vi "cost_complexity_pruning_path.vi"(8 "error in (no error)":errorcluster, 11 "Interface_cost_complexity_pruning_path in":refnum<class "Interface_cost_complexity_pruning_path.lvclass">) -> (0 "error out":errorcluster, 2 "out":cluster{"ccp_alphas":dbl[], "impurities":dbl[]}, 3 "Interface_cost_complexity_pruning_path out":refnum<class "Interface_cost_complexity_pruning_path.lvclass">)   [LabVIEW 2020, in "Interface_cost_complexity_pruning_path.lvclass"]
doc: "Compute the pruning path during Minimal Cost-Complexity Pruning."
uses:
  Interface_cost_complexity_pruning_path.lvclass
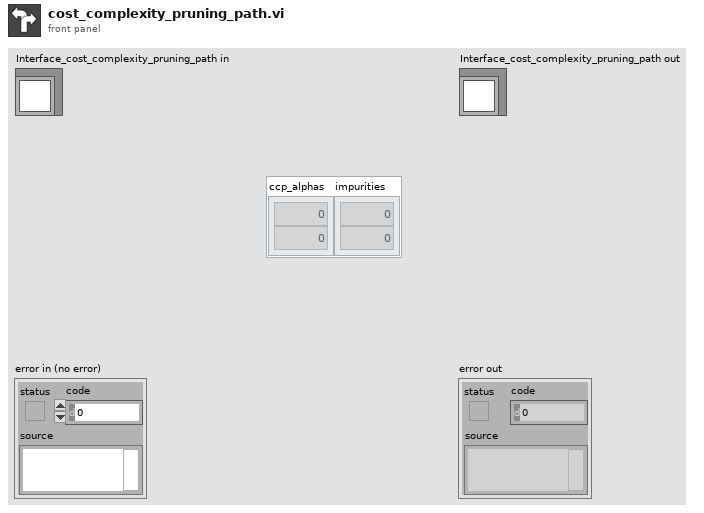
[diagram p1: front panel]
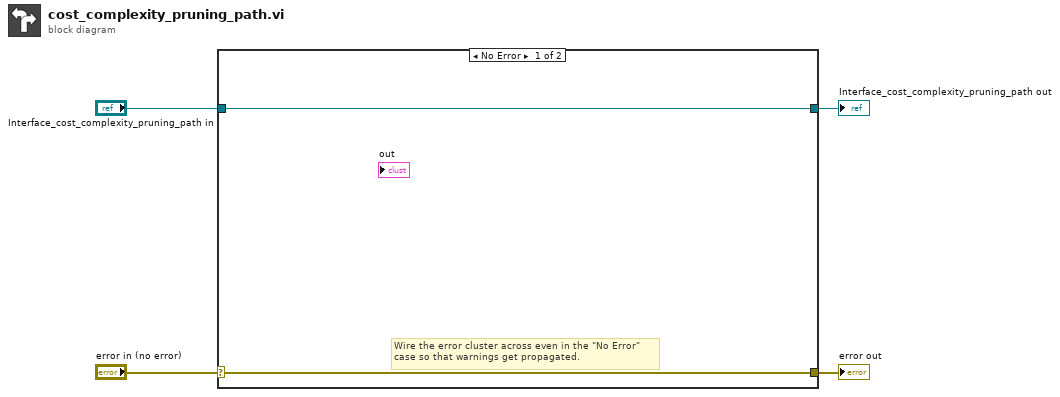
[diagram p0: block diagram]
diagram:
  n1 = case shown="No Error" "error in (no error)" {
    selector: "error in (no error)" -> [w5 w8]
    tunnel: [w5 w8] -> w3
    tunnel: [w6 w7] -> w1
    tunnel: "Interface_cost_complexity_pruning_path in" -> [w6 w7]
    frame No Error {
      # "Wire the error cluster across even in the \"No Error\"\ncase so that warnings get propagated."
    }
    frame Error {
    }
  }
  "error out" <- w3
  "Interface_cost_complexity_pruning_path out" <- w1
